vi "Read Spreadsheet Settings.vi"(11 "Selection":string) -> (3 "Autonomous Data":T1(array[cluster]))   [LabVIEW 2017]
uses:
  <vilib>/Utility/file.llb/Read Delimited Spreadsheet (DBL).vi
panel:
  out "error out":errorcluster
  out "all rows":dbl[][](array[numeric])
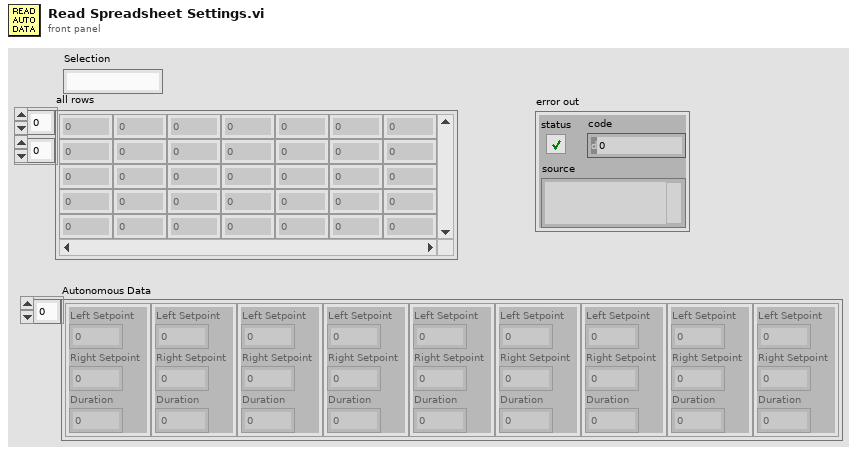
[diagram p1: front panel]
types:
  T1 = cluster{"Left Setpoint":dbl, "Right Setpoint":dbl, "Duration":dbl}[]
  T2 = cluster{"Left Setpoint":dbl, "Right Setpoint":dbl, "Duration":dbl}
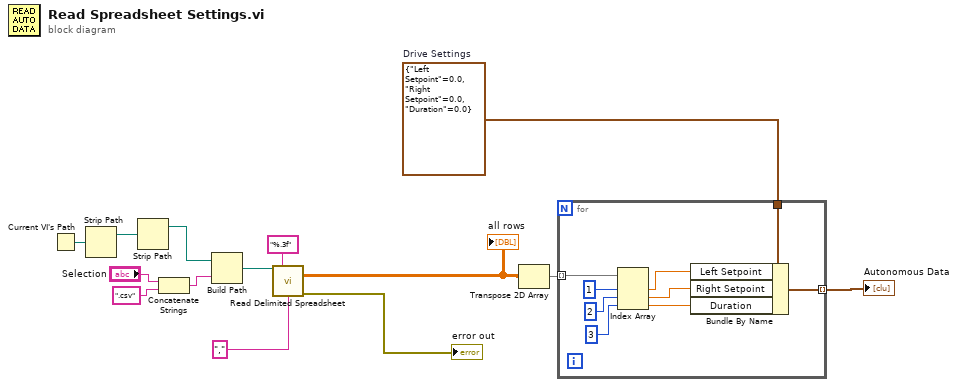
[diagram p0: block diagram]
diagram:
  w11 = T2 {"Left Setpoint"=0.0, "Right Setpoint"=0.0, "Duration"=0.0}  # Drive Settings
  n1 = Current VI's Path() -> (path=w3:path)
  n2 = Strip Path(path=w3) -> (stripped path=w2:path)  [unwired: 1 out]
  n3 = Strip Path(path=w2) -> (stripped path=w1:path)  [unwired: 1 out]
  n4 = Concatenate Strings("Selection", ".csv" ("string")) -> (w5:string)
  n5 = Build Path(base path=w1, name or relative path=w5) -> (appended path=w4:path)
  n6 = call-poly <vilib>:"Read Delimited Spreadsheet.vi"("file path (dialog if empty)"=w4, "format (%.3f)"="%.3f", "delimiter (\\t)"="," ("delimiter (\\t)")) -> ("all rows"=w8:dbl[][], "error out"=→"error out":errorcluster)  [unwired: 7 in, 4 out]
  "all rows" <- w8
  n7 = Transpose 2D Array(2D array=w8) -> (transposed array=w9:dbl[][])
  n8 = for {
    tunnel: w9 -> [w22] mode=indexing
    tunnel: w11 -> [w23]
    tunnel: [w18] -> w10 mode=indexing
    n9 = Index Array(array=w22, index #1=1 ("index"), index #2=2 ("index"), index #3=3 ("index")) -> (element #1=w21:dbl, element #2=w20:dbl, element #3=w19:dbl)
    n10 = Bundle By Name(cluster=w23, "Left Setpoint"=w21, "Right Setpoint"=w20, "Duration"=w19) -> (w18:T2)
  }
  "Autonomous Data" <- w10
